vi "FrameDown(SubVI).vi"(0 "input frame":string) -> (1 "size":string, 2 "id":string, 3 "sn":string, 4 "op":string, 6 "head":string, 8 "ob":string, 10 "data":string, 12 "len":dbl, 13 "reverse":string, 14 "chksum":string, 15 "result":string)   [LabVIEW 2012]
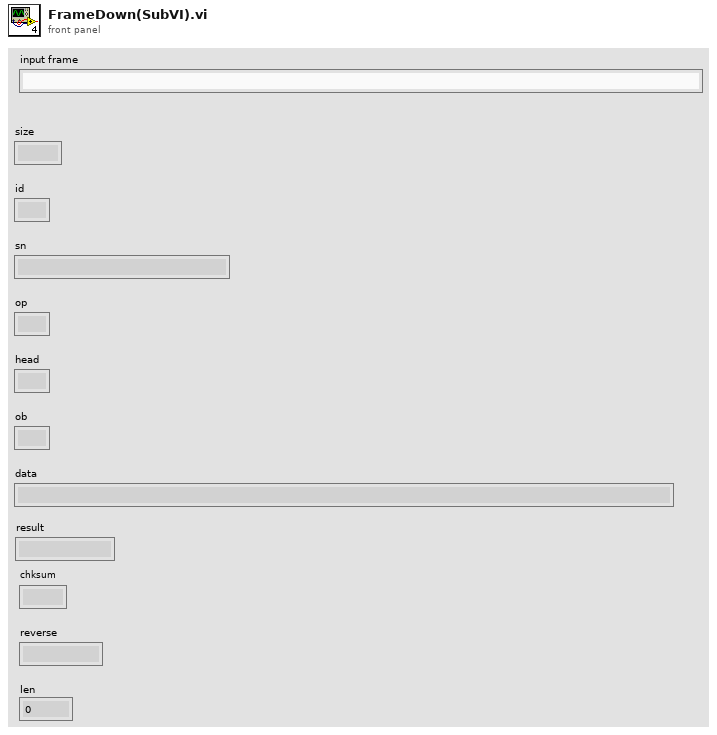
[diagram p1: front panel]
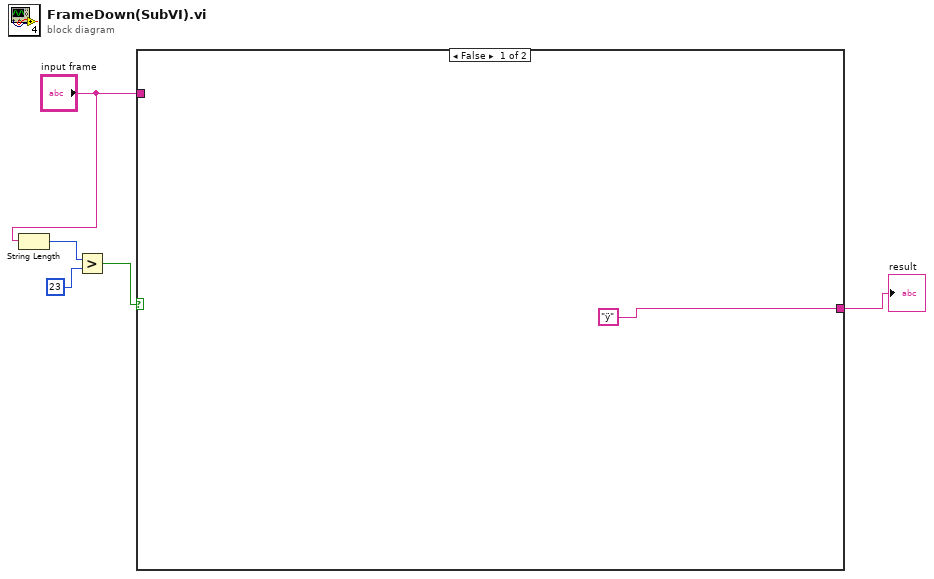
[diagram p0: block diagram]
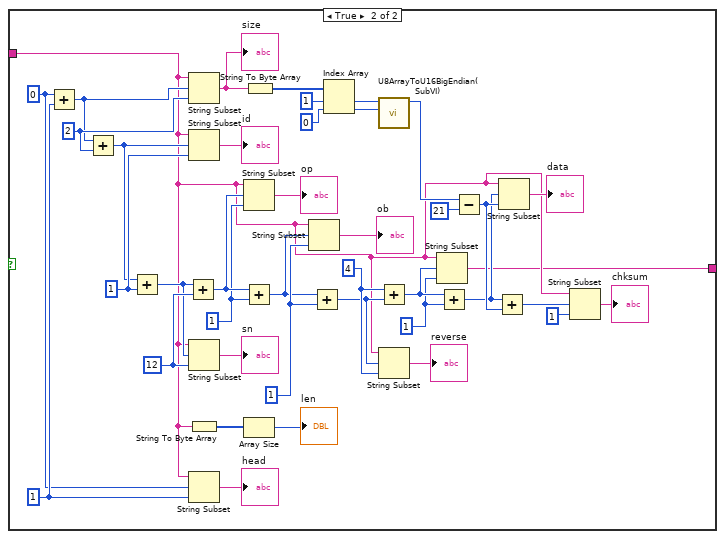
[diagram p2: hidden frame]
diagram:
  n1 = String Length(string="input frame") -> (length=w4:i32)
  n2 = Greater?(x=w4, y=23) -> (0:w2:bool)
  n3 = case shown="False" w2 {
    tunnel: "input frame" -> [_ w8]
    tunnel: ["ÿ" w7] -> w1
    frame False {
    }
    frame True {
      w10 = 1
      w31 = 4
      w26 = 1
      w23 = 1
      w22 = 12
      w20 = 1
      w40 = 2
      w16 = 1
      w15 = 0
      n4 = Add(x=w15, y=w16) -> (x+y=w39:i32)
      n5 = Add(x=w39, y=w40) -> (x+y=w19:i32)
      n6 = Add(x=w19, y=w20) -> (x+y=w21:i32)
      n7 = Add(x=w21, y=w22) -> (x+y=w24:i32)
      n8 = String Subset(string=w8, offset (0)=w39, length (rest)=w40) -> (substring=w41:string)
      "size" <- w41
      n9 = String Subset(string=w8, offset (0)=w19, length (rest)=w20) -> (substring=→"id":string)
      n10 = String Subset(string=w8, offset (0)=w21, length (rest)=w22) -> (substring=→"sn":string)
      n11 = String To Byte Array(string=w8) -> (unsigned byte array=w13:u8[])
      n12 = String Subset(string=w8, offset (0)=w15, length (rest)=w16) -> (substring=→"head":string)
      n13 = String Subset(string=w8, offset (0)=w24, length (rest)=w23) -> (substring=→"op":string)
      n14 = Add(x=w24, y=w23) -> (x+y=w25:i32)
      n15 = Array Size(array=w13) -> (size(s)=→"len":i32)
      n16 = String To Byte Array(string=w41) -> (unsigned byte array=w42:u8[])
      n17 = String Subset(string=w8, offset (0)=w25, length (rest)=w26) -> (substring=→"ob":string)
      n18 = Add(x=w25, y=w26) -> (x+y=w30:i32)
      n19 = Index Array(array=w42, index #1=1, index #2=0) -> (element #1=w45:u8, element #2=w46:u8)
      n20 = call "U8ArrayToU16BigEndian(SubVI).vi"("Numeric 7"=w46, "Numeric 6"=w45) -> ("Numeric 9"=w32:u16)  [unwired: 9 in]
      n21 = Add(x=w31, y=w30) -> (x+y=w11:i32)
      n22 = String Subset(string=w8, offset (0)=w30, length (rest)=w31) -> (substring=→"reverse":string)
      n23 = String Subset(string=w8, offset (0)=w11, length (rest)=w10) -> (substring=w7:string)
      n24 = Add(x=w11, y=w10) -> (x+y=w9:i32)
      n25 = Subtract(x=w32, y=21) -> (x-y=w35:i32)
      n26 = Add(x=w9, y=w35) -> (x+y=w36:i32)
      n27 = String Subset(string=w8, offset (0)=w9, length (rest)=w35) -> (substring=→"data":string)
      n28 = String Subset(string=w8, offset (0)=w36, length (rest)=1) -> (substring=→"chksum":string)
    }
  }
  "result" <- w1
